vi "Actor Core.vi"(8 "error in":errorcluster, 11 "Abstract Sensor in":refnum<class "Abstract Sensor.lvclass">) -> (0 "error out":errorcluster, 3 "Actor out":refnum<class "Actor.lvclass">)   [LabVIEW 2014, in "Abstract Sensor.lvlib" / "Abstract Sensor.lvclass"]
doc: "(<B>Filename</B>: Actor Framework.lvlib:Actor.lvclass:Actor Core.vi)\n\nReceives messages to the actor, reacts to them, and initiates any error handling that may shut the actor down.\n\nDescendant classes may override this VI to append parallel tasks for the actor to complete while it handles messages. Overrides use the Call Parent Method node."
uses:
  Abstract Sensor.lvclass
  <vilib>/ActorFramework/Actor/Actor.lvclass
  Generic Instrument/Generic Instrument.lvclass
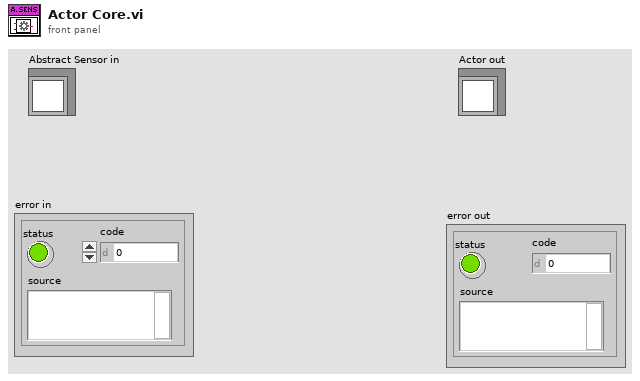
[diagram p1: front panel]
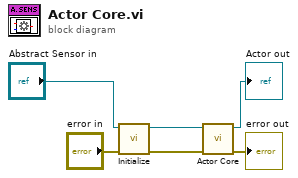
[diagram p0: block diagram]
diagram:
  n1 = call-dynamic "Initialize.vi"("error in (no error)"="error in", "Abstract Sensor in"="Abstract Sensor in") -> ("error out"=w1:errorcluster, "Abstract Sensor out"=w2:refnum<class "Abstract Sensor.lvclass">)  [unwired: 7 in, 1 out]
  n2 = call-parent "Actor Core.vi"("error in"=w1, "Actor in"=w2) -> ("error out"=→"error out":errorcluster, "Actor out"=→"Actor out":refnum<class "Actor.lvclass">)  [unwired: 8 in]
